vi "Signal Defect detection.vi"(8 "error in (no error)":errorcluster, 11 "Fiber Auto Collimation state data in":refnum<class "Fiber Auto Collimation state data.lvclass">) -> (0 "error out":errorcluster, 3 "Fiber Auto Collimation state data out":refnum<class "Fiber Auto Collimation state data.lvclass">)   [LabVIEW 2018]
uses:
  State data/Fiber Auto Collimation state data.lvclass
  <userlib>/nLight Tidbits/Logging/Controls/Logging type choice.ctl
  State data/Fiber Auto Collimation state data.lvclass/Fiber Auto Collimation state data.ctl
  State data/Add Changed data.vi
  <instrlib>/nLight Instruments/Beam Profiler/Beam Profiler.lvclass
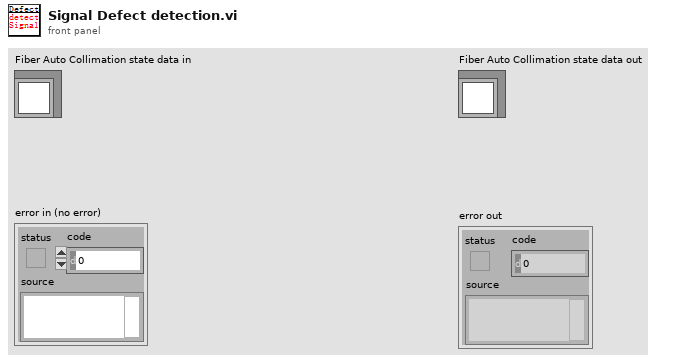
[diagram p1: front panel]
types:
  T1 = typedef "Logging type choice.ctl" = enum16{"No log type selected", "Testing start/stop", "Test progress", "Station startup/shutdown", "Station config change", "Recipe load/change", "Inventory transaction", "Instrument", "Debug"}
  T2 = typedef "Test Parameters.ctl" = cluster{"Start position":dbl, "Peak Resp_min":dbl, "Circularity_min":dbl, "Beam Size Target":dbl, "Beam Size Percentage ":dbl, "Collimation Steps Data Path":string, "Collimation Data Path":string, "Defect detection Image Path":string, "Save Collimation Steps Data Enable":bool, "Defect detection Enable":bool, "Stop position":dbl}
  T3 = typedef "IMAQ Image.ctl" = refnum<image>
  T4 = typedef "VBAIInterface.ctl" = refnum<k21>
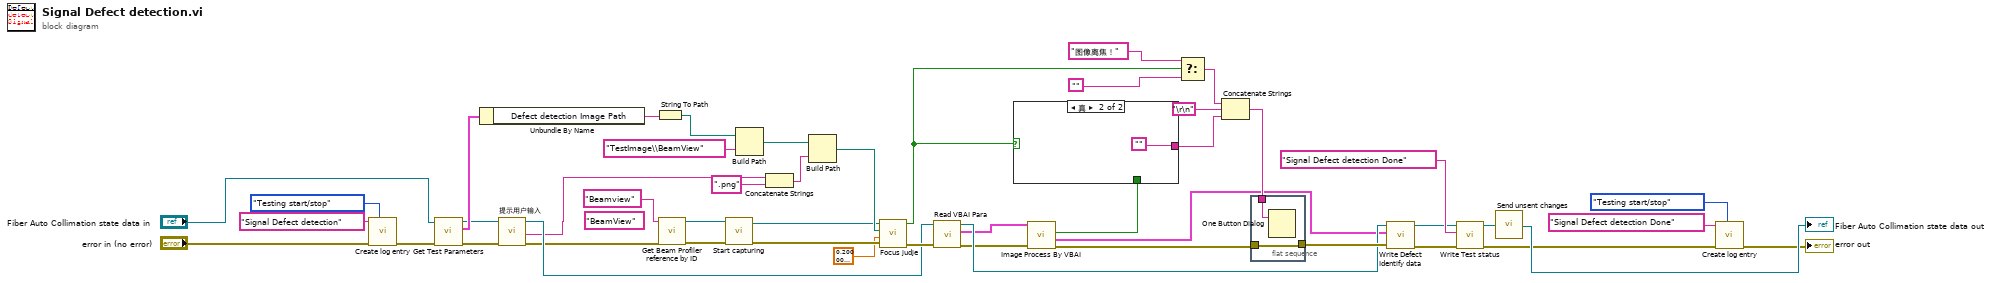
[diagram p0: block diagram]
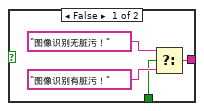
[diagram p2: hidden frame]
diagram:
  (unwired) "BeamView"
  n1 = call <userlib>:"Create log entry.vi"("Logging type choice"=Logging_type_choice."Testing start/stop", "error in (no error)"="error in (no error)", "Brief log entry"="Signal Defect detection") -> ("error out"=w24:errorcluster)  [unwired: 8 in]
  n2 = call "Get Test Parameters.vi"("error in (no error)"=w24, "Fiber Auto Collimation state data in"="Fiber Auto Collimation state data in") -> ("error out"=w20:errorcluster, "TestParameters"=w47:T2, "Fiber Auto Collimation state data out"=w21:refnum<class "Fiber Auto Collimation state data.lvclass">)  [unwired: 7 in]
  n3 = Unbundle By Name(w47) -> ("Defect detection Image Path"=w40:string)
  n4 = call "提示用户输入"("error in (no error)"=w20) -> ("SN"=w19:string, "error out"=w7:errorcluster)  [unwired: 16 in, 1 out]
  n5 = String To Path(string=w40) -> (path=w45:path)
  n6 = call <instrlib>:"Get Beam Profiler reference by ID.vi"("error in (no error)"=w7, "Identifier"="Beamview") -> ("error out"=w9:errorcluster, "Beam Profiler out"=w8:refnum<class "Beam Profiler.lvclass">)  [unwired: 8 in]
  n7 = call-dynamic "Start capturing.vi"("error in (no error)"=w9, "Beam Profiler in"=w8) -> ("error out"=w6:errorcluster, "Beam Profiler out"=w3:refnum<class "Beam Profiler.lvclass">)  [unwired: 8 in]
  n8 = Build Path(base path=w45, name or relative path="TestImage\\BeamView") -> (appended path=w42:path)
  n9 = Concatenate Strings(w19, ".png" ("string")) -> (w43:string)
  n10 = Build Path(base path=w42, name or relative path=w43) -> (appended path=w4:path)
  n11 = call "Focus judje.vi"("error in"=w6, "Standard Variation Limit"=sgl 0.2, "File Path"=w4, "Beam Profiler in"=w3) -> ("error out"=w41:errorcluster, "离焦？"=w10:bool)  [unwired: 5 in, 1 out]
  n12 = call "Read VBAI Para.vi"("error in (no error)"=w41, "Fiber Auto Collimation state data in"=w21) -> ("error out"=w14:errorcluster, "VBAI"=w15:cluster{"New Image":T3, "VBAI Session Out":T4}, "Fiber Auto Collimation state data out"=w34:refnum<class "Fiber Auto Collimation state data.lvclass">)  [unwired: 7 in]
  n13 = call "Image Process By VBAI.vi"("error in"=w14, "VBAI"=w15) -> ("error out"=w11:errorcluster, "Defect identify data"=w12:cluster{"Image":T3, "Measure Report":string}, "Result"=w13:bool)  [unwired: 4 in, 3 out]
  n14 = case shown="真" w10 {
    tunnel: [w49 ""] -> w29
    tunnel: w13 -> [w48 _]
    frame False {
      n15 = Select(t="图像识别无脏污！", s=w48, f="图像识别有脏污！") -> (s? t:f=w49:string)
    }
    frame True {
    }
  }
  n16 = Select(t="图像离焦！", s=w10, f="") -> (s? t:f=w31:string)
  n17 = Concatenate Strings(w31, "\r\n", w29) -> (w33:string)
  n18 = flat-sequence {
    tunnel: w11 -> [w54]
    tunnel: [w54] -> w35
    tunnel: w33 -> [w53]
    frame #0 {
      n19 = One Button Dialog(message=w53) -> ()  [unwired: 1 in, 1 out]
    }
  }
  n20 = call "Write Defect Identify data.vi"("error in (no error)"=w35, "Defect Identify data"=w12, "Fiber Auto Collimation state data in"=w34) -> ("error out"=w37:errorcluster, "Fiber Auto Collimation state data out"=w36:refnum<class "Fiber Auto Collimation state data.lvclass">)  [unwired: 7 in]
  n21 = call "Write Test status.vi"("error in (no error)"=w37, "Test status"="Signal Defect detection Done", "Fiber Auto Collimation state data in"=w36) -> ("error out"=w17:errorcluster, "Fiber Auto Collimation state data out"=w39:refnum<class "Fiber Auto Collimation state data.lvclass">)  [unwired: 7 in]
  n22 = call "Send unsent changes.vi"("Fiber Auto Collimation state data in"=w39) -> ("Fiber Auto Collimation state data out"=→"Fiber Auto Collimation state data out":refnum<class "Fiber Auto Collimation state data.lvclass">)  [unwired: 1 in]
  n23 = call <userlib>:"Create log entry.vi"("Logging type choice"=Logging_type_choice."Testing start/stop", "error in (no error)"=w17, "Brief log entry"="Signal Defect detection Done") -> ("error out"=→"error out":errorcluster)  [unwired: 8 in]
